vi "Destructor.vi"(8 "ErrorIn":errorcluster, 11 "ObjectIn":refnum<class "DotNETCam.lvclass">) -> (0 "ErrorOut":errorcluster, 3 "ObjectOut":refnum<class "DotNETCam.lvclass">)   [LabVIEW 2021, in "DotNETCam.lvclass"]
uses:
  DotNETCam.lvclass
  DotNETCam.lvclass/DotNETCam.ctl
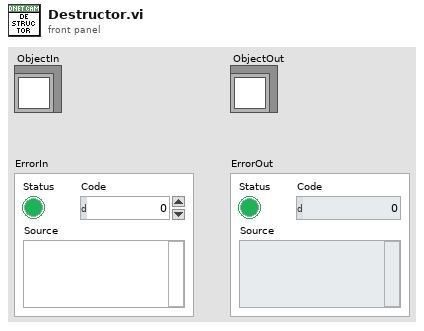
[diagram p1: front panel]
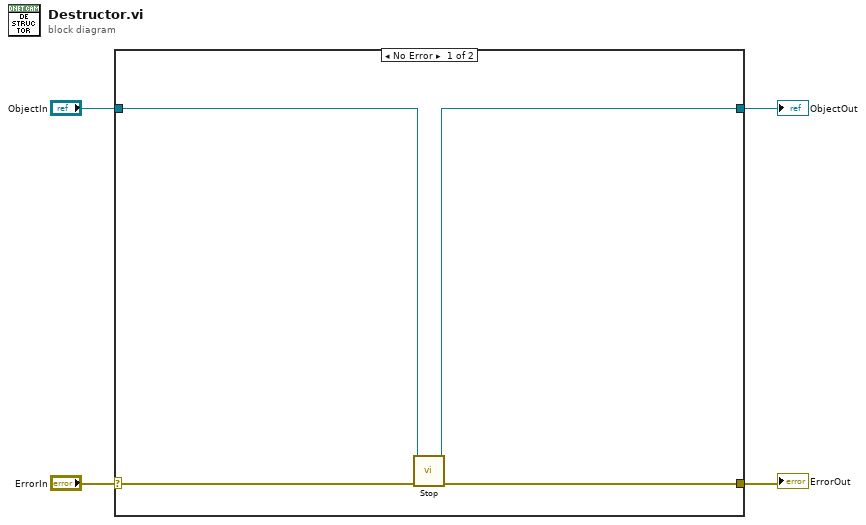
[diagram p0: block diagram]
diagram:
  n1 = case shown="No Error" "ErrorIn" {
    selector: "ErrorIn" -> [w8 w10]
    tunnel: [w7 w10] -> w3
    tunnel: [w5 w9] -> w1
    tunnel: "ObjectIn" -> [w6 w9]
    frame No Error {
      n2 = call-dynamic "Stop.vi"("ErrorIn"=w8, "DotNETCamIn"=w6) -> ("ErrorOut"=w7:errorcluster, "DotNETCamOut"=w5:refnum<class "DotNETCam.lvclass">)  [unwired: 8 in]
    }
    frame Error {
    }
  }
  "ErrorOut" <- w3
  "ObjectOut" <- w1
